vi "Set Log File Location.vi"(8 "error in":errorcluster, 9 "timestamp file name":bool=TRUE, 10 "directory parts":string[](array[string]), 11 "log file in":T1 format="%.0x") -> (0 "error out":errorcluster, 2 "sample path":path, 3 "log file out":T1 format="%.0x")   [LabVIEW 2027, in "Embedded Data Logger Scripting.lvlib"]
uses:
  Embedded Data Logger Scripting.lvlib
  <vilib>/NI VeriStand/Custom Device API/Custom Device Item Ref.ctl
  Shared/Constants.vi
  <vilib>/NI VeriStand/Custom Device API/Set Item Property (String Array).vi
  <vilib>/NI VeriStand/Custom Device API/Set Item Property (Boolean).vi
  <vilib>/NI VeriStand/Custom Device API/Custom Device API.lvlib
  Shared/Embedded Data Logger Shared.lvlib
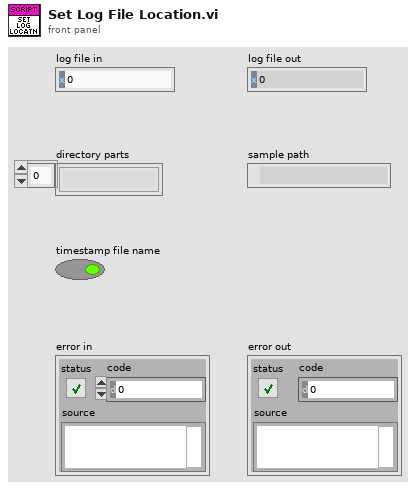
[diagram p1: front panel]
types:
  T1 = typedef "Custom Device API.lvlib/Custom Device Item Ref.ctl" = u64
  T2 = typedef "Custom Device API.lvlib/Custom Device Item Info.ctl" = cluster{"Name":string, "Is Channel":bool, "GUID":string, "Is Waveform":bool}
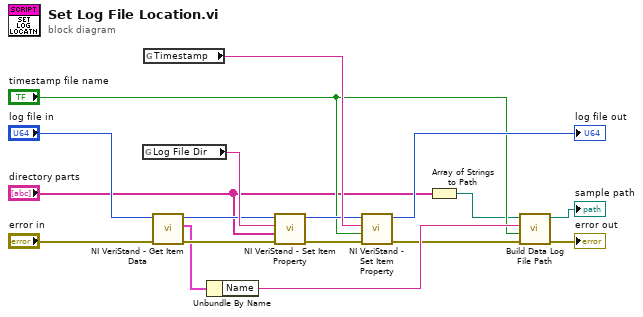
[diagram p0: block diagram]
diagram:
  n1 = global read "Constants.vi" "Log File Dir"() -> (w16:string)
  n2 = global read "Constants.vi" "Timestamp"() -> (w17:string)
  n3 = call <vilib>:"NI VeriStand - Get Item Data.vi"("error in (no error)"="error in", "Item Ref in"="log file in") -> ("error out"=w9:errorcluster, "Item Info"=w8:T2, "Item Ref out"=w10:T1)  [unwired: 7 out]
  n4 = Unbundle By Name(w8) -> ("Name"=w7:string)
  n5 = call-poly <vilib>:"NI VeriStand - Set Item Property.vi"("error in (no error)"=w9, "Value"="directory parts", "Property Name"=w16, "Item Ref in"=w10) -> ("error out"=w14:errorcluster, "Item Ref out"=w13:T1)  [unwired: 6 out]
  n6 = call-poly <vilib>:"NI VeriStand - Set Item Property.vi"("error in (no error)"=w14, "Value"="timestamp file name", "Property Name"=w17, "Item Ref in"=w13) -> ("error out"=w6:errorcluster, "Item Ref out"=→"log file out":T1)  [unwired: 6 out]
  n7 = Array of Strings to Path(0:"directory parts") -> (2:w2:path)  [unwired: 1 in]
  n8 = call "Build Data Log File Path.vi"("error in (no error)"=w6, "Timestamp"="timestamp file name", "Name"=w7, "Log File Directory"=w2) -> ("error out"=→"error out":errorcluster, "appended path"=→"sample path":path)  [unwired: 6 in]
